vi "Test.vi"(8 "error constant":errorcluster, 10 "Array":T2(array[cluster]), 11 "file path (dialog if empty)":path) -> (0 "error out":errorcluster)   [LabVIEW 2019]
uses:
  ADC_CTRL.ctl
  <vilib>/Utility/file.llb/Write Delimited Spreadsheet (string).vi
panel:
  out "ADC":T1
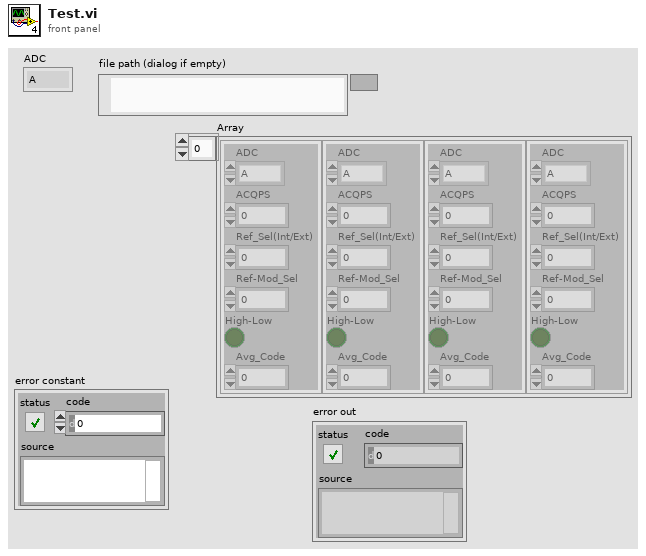
[diagram p1: front panel]
types:
  T1 = typedef "ADC_CTRL.ctl" = enum16{"A", "B", "C"}
  T2 = cluster{"ADC":T1, "ACQPS":u16, "Ref_Sel(Int/Ext)":u16, "Ref-Mod_Sel":u16, "High-Low":bool, "Avg_Code":dbl}[]
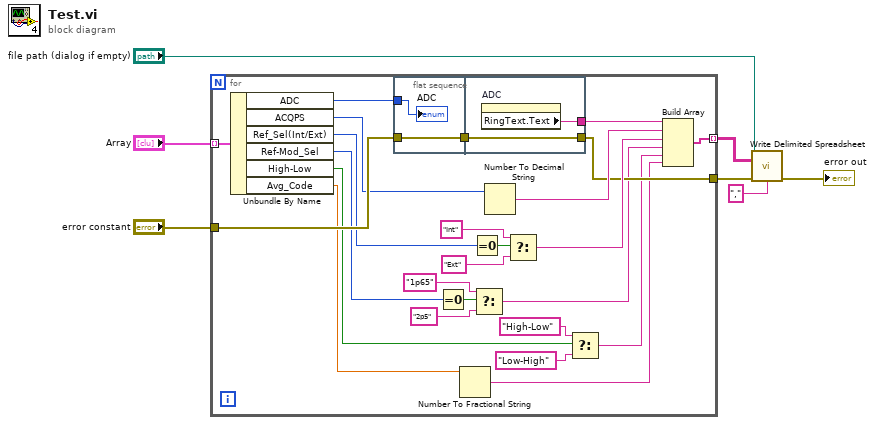
[diagram p0: block diagram]
diagram:
  n1 = for {
    tunnel: "Array" -> [w32] mode=indexing
    tunnel: "error constant" -> [w31]
    tunnel: [w16] -> w6
    tunnel: [w15] -> w4 mode=indexing
    n2 = Unbundle By Name(w32) -> ("ADC"=w29:T1, "ACQPS"=w28:u16, "Ref_Sel(Int/Ext)"=w21:u16, "Ref-Mod_Sel"=w17:u16, "High-Low"=w8:bool, "Avg_Code"=w13:dbl)
    n3 = flat-sequence {
      tunnel: w31 -> [w34]
      tunnel: [w34] -> w30
      tunnel: w29 -> [w33]
      tunnel: [w36] -> w24
      tunnel: [w35] -> w16
      tunnel: w30 -> [w35]
      frame #0 {
        "ADC" <- w33
      }
      frame #1 {
        n4 = property on="ADC" class="Enum (strict)"() -> ("RingText.Text"=w36:string)  [unwired: 2 in, 2 out]
      }
    }
    n5 = Equal To 0?(x=w17) -> (x = 0?=w18:bool)
    n6 = Number To Fractional String(number=w13) -> (F-format string=w11:string)  [unwired: 3 in]
    n7 = Equal To 0?(x=w21) -> (x = 0?=w27:bool)
    n8 = Select(t="1p65", s=w18, f="2p5") -> (s? t:f=w14:string)
    n9 = Number To Decimal String(number=w28) -> (decimal integer string=w23:string)  [unwired: 1 in]
    n10 = Select(t="Int", s=w27, f="Ext") -> (s? t:f=w22:string)
    n11 = Select(t="High-Low", s=w8, f="Low-High") -> (s? t:f=w10:string)
    n12 = Build Array(w24, w23, w22, w14, w10, w11) -> (w15:string[])
  }
  n13 = call-poly <vilib>:"Write Delimited Spreadsheet.vi"("file path (dialog if empty)"="file path (dialog if empty)", "2D data"=w4, "error in (no error)"=w6, "delimiter (\\t)"="," ("delimiter (\\t)")) -> ("error out"=→"error out":errorcluster)  [unwired: 10 in, 1 out]
